vi "Consumer.vi"(8 "error in (no error)":errorcluster, 9 "Data":variant, 10 "Case ID":string, 11 "uService Template in":refnum<class "Dummy.lvclass">) -> (0 "error out":errorcluster, 3 "uService Template out":refnum<class "Dummy.lvclass">)   [LabVIEW 2020, in "Dummy.lvlib" / "Dummy.lvclass"]
uses:
  Dummy.lvclass
  Dummy Consumer Case Selector.ctl
  TALOS/TALOS_PPL.lvlibp/Father of all uServices/Father of all uServices/Father of all uServices.lvclass
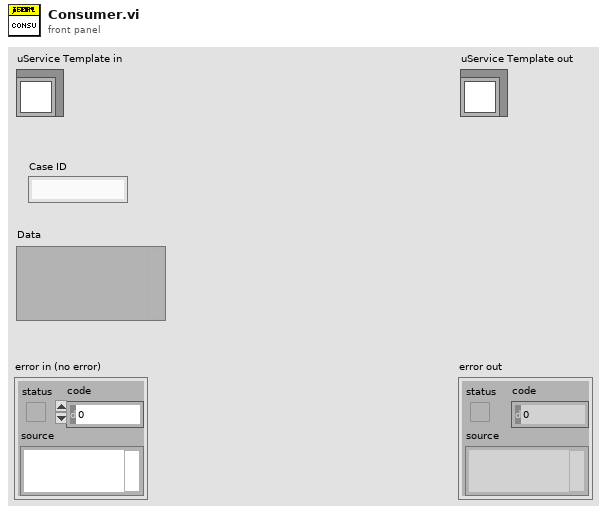
[diagram p1: front panel]
types:
  T1 = typedef "Dummy.lvlib/Dummy.lvclass/Dummy Consumer Case Selector.ctl" = enum16{""}
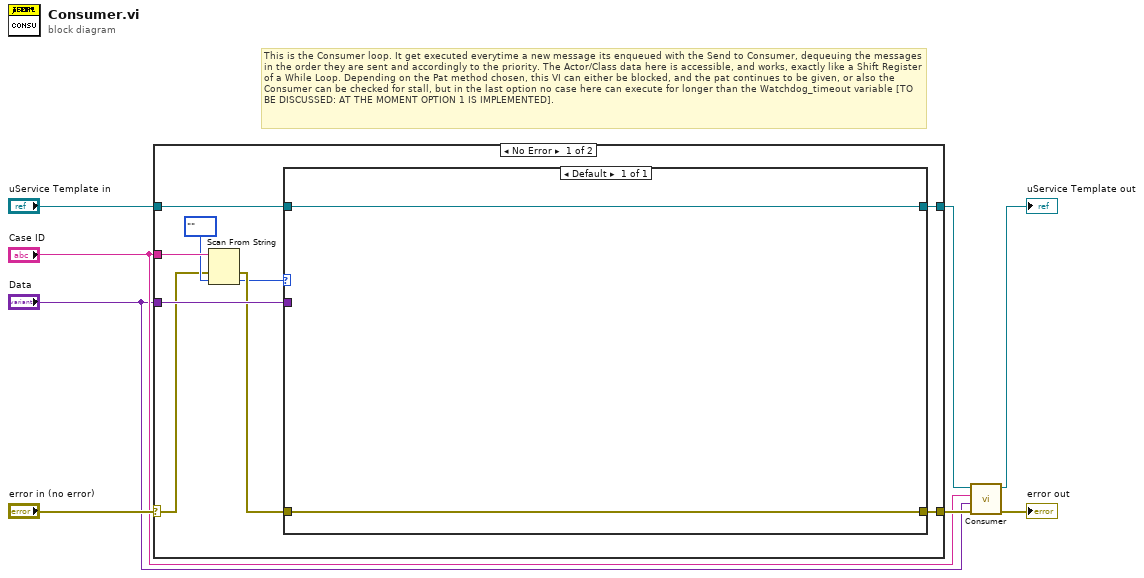
[diagram p0: block diagram]
diagram:
  # "This is the Consumer loop. It get executed everytime a new message its enqueued with the Send to Consumer, dequeuing the messages in the order they are sent and accordingly to the priority. The Actor/Class data here is accessible, and works, exactly like a Shift Register of a While Loop. Depending on the Pat method chosen, this VI can either be blocked, and the pat continues to be given, or also the Consumer can be checked for stall, but in the last option no case here can execute for longer than the Watchdog_timeout variable [TO BE DISCUSSED: AT THE MOMENT OPTION 1 IS IMPLEMENTED]."
  n1 = case shown="No Error" "error in (no error)" {
    selector: "error in (no error)" -> [w11 w20]
    tunnel: [w16 w21] -> w3
    tunnel: "uService Template in" -> [w17 w21]
    tunnel: [w14 w20] -> w6
    tunnel: "Case ID" -> [w13 _]
    tunnel: "Data" -> [w15 _]
    frame No Error {
      n2 = Scan From String(input string=w13, error in=w11, default 1=Dummy_Consumer_Case_Selector."" ("Consumer Case Selector")) -> (error out=w10:errorcluster, output 1=w9:T1)  [unwired: 2 in, 2 out]
      n3 = case shown="Default" w9 {
        tunnel: w17 -> [w19]
        tunnel: [w19] -> w16
        tunnel: w15 -> [_]
        tunnel: [w18] -> w14
        tunnel: w10 -> [w18]
        frame Default {
        }
      }
    }
    frame Error {
    }
  }
  n4 = call-parent "Consumer.vi"("error in (no error)"=w6, "Data"="Data", "Case ID"="Case ID", "uService Template in"=w3) -> ("error out"=→"error out":errorcluster, "uService Template out"=→"uService Template out":refnum<class "Dummy.lvclass">)  [unwired: 6 in]
